vi "OPC client side test.vi"() -> ()   [LabVIEW 2015]
uses:
  <vilib>/OPCUA/client/Write Double.vi
  <vilib>/OPCUA/NI OPC UA Client.lvlib
panel:
  out "status":u32(ring) items=["Good"=0, "Bad_AttributeIdInvalid"=2153906176, "Bad_BrowseDirectionInvalid"=2152529920, "Bad_BrowseNameInvalid"=2153775104, "Bad_ContentFilterInvalid"=2152202240, "Bad_ContinuationPointInvalid"=2152333312, "Bad_DataEncodingInvalid"=2151153664, "Bad_DataEncodingUnsupported"=2151219200, "Bad_EventFilterInvalid"=2152136704, "Bad_FilterNotAllowed"=2152005632, "Bad_FilterOperandInvalid"=2160132096, "Bad_HistoryOperationInvalid"=2154889216, "Bad_HistoryOperationUnsupported"=2154954752, "Bad_IndexRangeInvalid"=2151022592, "Bad_IndexRangeNoData"=2151088128, "Bad_MonitoredItemFilterInvalid"=2151874560, "Bad_MonitoredItemFilterUnsupported"=2151940096, "Bad_MonitoredItemIdInvalid"=2151809024, "Bad_MonitoringModeInvalid"=2151743488, "Bad_NoCommunication"=2150694912, "Bad_NoContinuationPoints"=2152398848, "Bad_NodeClassInvalid"=2153709568, "Bad_NodeIdInvalid"=2150825984, "Bad_NodeIdUnknown"=2150891520, "Bad_NoDeleteRights"=2154364928, "Bad_NodeNotInView"=2152595456, "Bad_NotFound"=2151546880, "Bad_NotImplemented"=2151677952, "Bad_NotReadable"=2151284736, "Bad_NotSupported"=2151481344, "Bad_NotWritable"=2151350272, "Bad_ObjectDeleted"=2151612416, "Bad_OutOfRange"=2151415808, "Bad_ReferenceTypeIdInvalid"=2152464384, "Bad_SourceNodeIdInvalid"=2154037248, "Bad_StructureMissing"=2152071168, "Bad_TargetNodeIdInvalid"=2154102784, "Bad_TypeDefinitionInvalid"=2153971712, "Bad_TypeMismatch"=2155085824, "Bad_WaitingForInitialData"=2150760448]
  out "browse result":T1(array[cluster])
  out "error out":errorcluster
  out "OPC UA change events":dbl(graph)
  in  "stop":bool
  in  "OPC UA link":dbl=1000.0
  in  "SV link":dbl=1000.0
  in  "server endpoint URL":string="opc.tcp://192.168.1.50:4840"
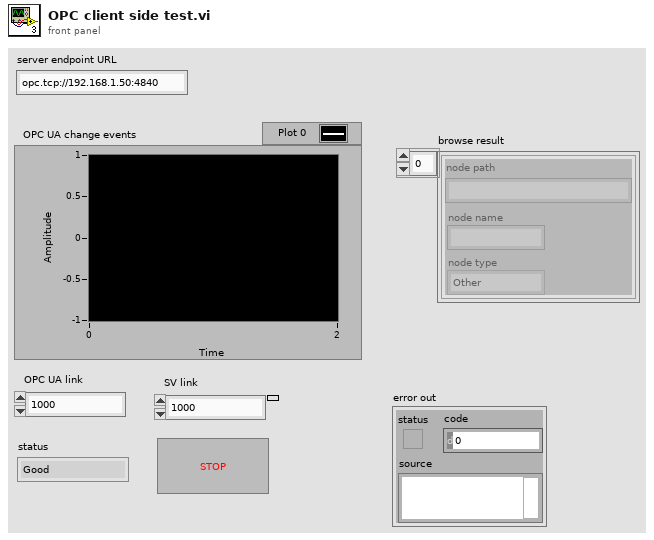
[diagram p1: front panel]
types:
  T1 = cluster{"node path":string, "node name":string, "node type":enum32{"Other", "Folder", "Item/Property"}}[]
  T2 = cluster{"message mode":enum16{"None", "Sign", "Sign and Encrypt"}, "security":enum16{"Basic256", "Basic128Rsa15"}}
  T3 = cluster{"Item URL":string, "Item Value":variant, "Timestamp":timestamp, "DataType":u32, "status code":u32}[]
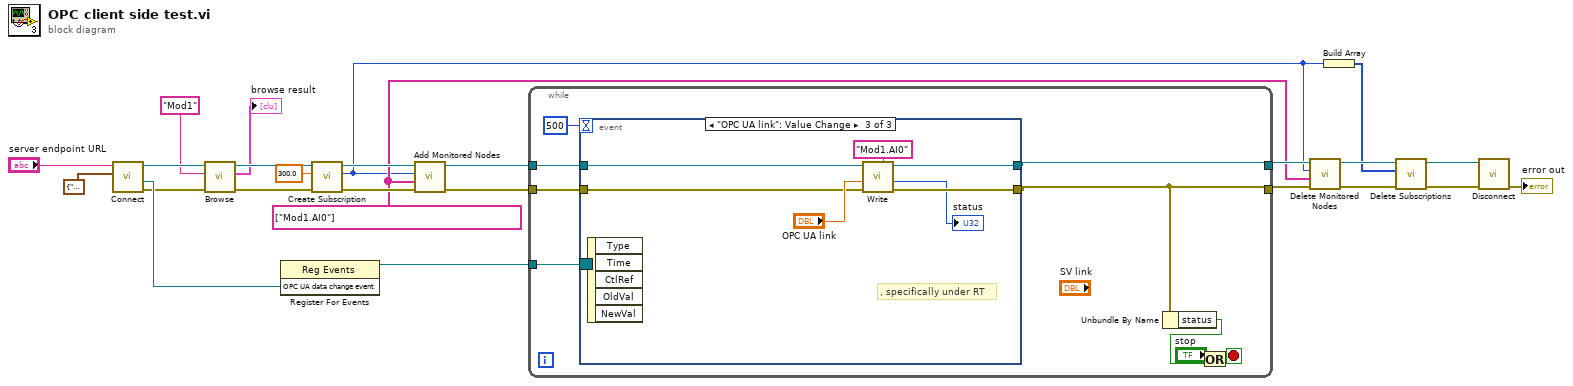
[diagram p0: block diagram]
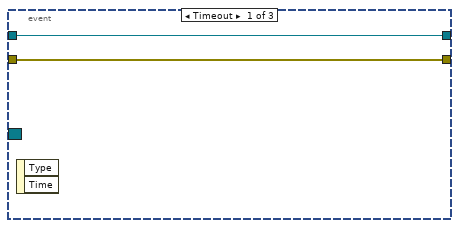
[diagram p2: hidden frame]
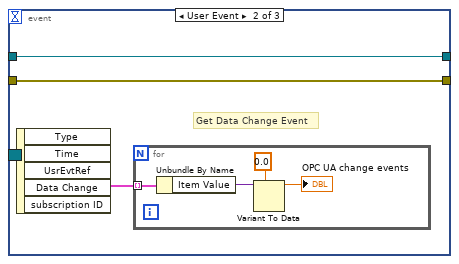
[diagram p3: hidden frame]
diagram:
  w10 = string[] ["Mod1.AI0"] ("array of node path")
  n1 = call <vilib>:"Connect.vi"("security policy"=T2 {"message mode"=enum."None", "security"=enum."Basic256"}, "server endpoint URL"="server endpoint URL") -> ("error out"=w6:errorcluster, "OPC UA data change event"=w21:refnum<user-event>, "OPC UA client refnum out"=w5:refnum<k21>)  [unwired: 7 in]
  n2 = call <vilib>:"Browse.vi"("error in (no error)"=w6, "node path"="Mod1", "OPC UA client refnum in"=w5) -> ("error out"=w1:errorcluster, "browse result"=→"browse result":T1, "OPC UA client refnum out"=w4:refnum<k21>)  [unwired: 5 in, 1 out]
  n3 = register-events(w21) -> (reference out=w20:refnum<event-registration>)  [unwired: 2 in, 1 out]
  n4 = call <vilib>:"Create Subscription.vi"("error in (no error)"=w1, "update rate (1000 ms)"=300.0, "OPC UA client refnum in"=w4) -> ("error out"=w22:errorcluster, "subscription ID out"=w9:u32, "OPC UA client refnum out"=w23:refnum<k21>)  [unwired: 6 in]
  n5 = call <vilib>:"Add Monitored Nodes.vi"("error in (no error)"=w22, "array of node path"=w10, "subscription ID in"=w9, "OPC UA client refnum in"=w23) -> ("error out"=w18:errorcluster, "OPC UA client refnum out"=w19:refnum<k21>)  [unwired: 5 in, 1 out]
  n6 = while {
    tunnel: w20 -> [w34]
    tunnel: w19 -> [w32]
    tunnel: w18 -> [w31]
    tunnel: [w26] -> w16
    tunnel: [w27] -> w17
    stop <- w29 stop-if-true
    n7 = event shown="[2] \"OPC UA link\": Value Change" {
      selector: w34 -> [_ _ _]
      dyn-events: _ -> [_ _ _]
      timeout: 500 -> [_ _ _]
      tunnel: w32 -> [w36 w39 w46]
      tunnel: w31 -> [w35 w38 w45]
      tunnel: [w36 w39 w48] -> w27
      tunnel: [w35 w38 w47] -> w26
      event Timeout {
        n8 = event-data() -> ()  [unwired: 1 in, 2 out]
      }
      event User Event {
        # "Get Data Change Event"
        n9 = event-data() -> ("Data Change"=w37:T3)  [unwired: 1 in, 4 out]
        n10 = for {
          tunnel: w37 -> [w43] mode=indexing
          n11 = Unbundle By Name(w43) -> ("Item Value"=w42:variant)
          n12 = Variant To Data(type=0.0, Variant=w42) -> (data=→"OPC UA change events":dbl)  [unwired: 1 in, 1 out]
        }
      }
      event "OPC UA link": Value Change {
        # ", specifically under RT"
        n13 = event-data() -> ()  [unwired: 1 in, 5 out]
        n14 = call-poly <vilib>:"Write.vi"("error in (no error)"=w45, "value"="OPC UA link", "node path"="Mod1.AI0", "OPC UA client refnum in"=w46) -> ("error out"=w47:errorcluster, "status"=→"status":u32, "OPC UA client refnum out"=w48:refnum<k21>)  [unwired: 5 in]
      }
    }
    n15 = Unbundle By Name(w26) -> ("status"=w28:bool)
    n16 = Or(x="stop", y=w28) -> (x .or. y?=w29:bool)
  }
  n17 = call <vilib>:"Delete Monitored Nodes.vi"("error in (no error)"=w16, "array of node path"=w10, "subscription ID in"=w9, "OPC UA client refnum in"=w17) -> ("error out"=w14:errorcluster, "OPC UA client refnum out"=w15:refnum<k21>)  [unwired: 4 in, 2 out]
  n18 = Build Array(w9) -> (w8:u32[])
  n19 = call <vilib>:"Delete Subscriptions.vi"("error in (no error)"=w14, "array of subscription ID"=w8, "OPC UA client refnum in"=w15) -> ("error out"=w12:errorcluster, "OPC UA client refnum out"=w13:refnum<k21>)  [unwired: 6 in, 1 out]
  n20 = call <vilib>:"Disconnect.vi"("error in (no error)"=w12, "OPC UA client refnum in"=w13) -> ("error out"=→"error out":errorcluster)  [unwired: 9 in]
